vi "Limit Specification By Formula.vi"   [LabVIEW 2020, in "NI_MAPro.lvlib"]
doc: "Creates a continuous or segmented mask in the time domain or in the frequency domain. You can use different instances of this VI to create multiple limits. Wire data to the <B>Specification Cluster</B> input to determine the polymorphic instance to use or manually select the instance."
uses:
  NI_MAPro.lvlib
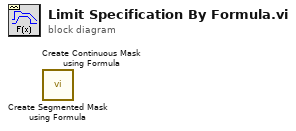
[diagram p0: block diagram]
diagram:
  n1 = call "Create Segmented Mask using Formula.vi"() -> ()  [unwired: 5 in, 2 out]
  n2 = call "Create Continuous Mask using Formula.vi"() -> ()  [unwired: 5 in, 2 out]
